vi "Elevator PID.vi"(2 "error in":errorcluster, 3 "PID gains":T1={"proportional gain (Kc)"=0.01, "integral time (Ti, min)"=0.0, "derivative time (Td, min)"=0.0}, 4 "Position":dbl format="%.2f") -> (0 "error out":errorcluster, 1 "Motor Output":dbl format="%.2f")   [LabVIEW 2018]
uses:
  <vilib>/addons/control/pid/pid.llb/PID (DBL).vi
  <vilib>/addons/control/pid/NI_PID_pid.lvlib
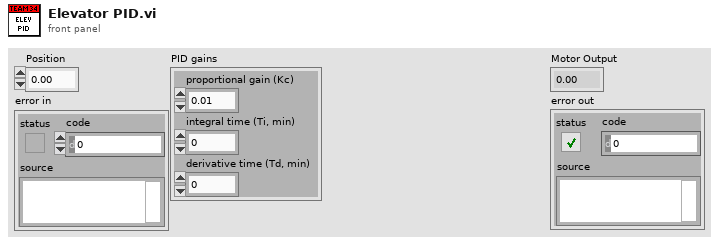
[diagram p1: front panel]
types:
  T1 = cluster{"proportional gain (Kc)":dbl, "integral time (Ti, min)":dbl, "derivative time (Td, min)":dbl}
  T2 = typedef "WPI_EncoderDevRef.ctl" = cluster{"DevStatus":errorcluster, "EncoderIndex":T3, "CounterIndex":T4, "DistancePerCount":dbl, "Decoding Type":T5}
  T3 = typedef "FPGA_EncoderIdx.ctl" = enum8{"Enc 0", "Enc 1", "Enc 2", "Enc 3", "Enc 4", "Enc 5", "Enc 6", "Enc 7", "Invalid"}
  T4 = typedef "FPGA_CounterCtrSystemIndex.ctl" = enum8{"Ctr 0", "Ctr 1", "Ctr 2", "Ctr 3", "Ctr 4", "Ctr 5", "Ctr 6", "Ctr 7", "Invalid"}
  T5 = typedef "WPI_EncoderType.ctl" = enum16{"1x", "2x", "4x"}
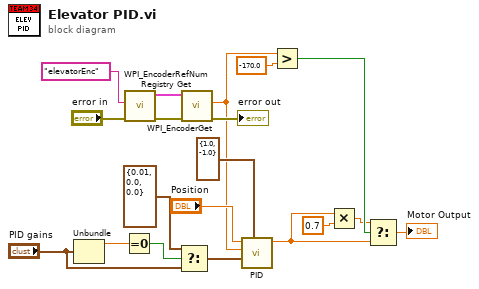
[diagram p0: block diagram]
diagram:
  n1 = Unbundle("PID gains") -> ("proportional gain (Kc)"=w13:dbl)  [unwired: 2 out]
  n2 = Equal To 0?(x=w13) -> (x = 0?=w10:bool)
  n3 = call <vilib>:"WPI_EncoderRefNum Registry Get.vi"("error in (no error)"="error in", "refnum name"="elevatorEnc") -> ("error out"=w15:errorcluster, "EncoderDevRef"=w18:T2)  [unwired: 8 in]
  n4 = Select(t=T1 {"proportional gain (Kc)"=0.01, "integral time (Ti, min)"=0.0, "derivative time (Td, min)"=0.0} ("PID gains"), s=w10, f="PID gains") -> (s? t:f=w11:T1)
  n5 = call <vilib>:"WPI_EncoderGet.vi"("error in (no error)"=w15, "EncoderDevRef"=w18) -> ("error out"=→"error out":errorcluster, "Distance"=w7:dbl)  [unwired: 4 in, 4 out]
  n6 = call-poly <vilib>:"PID.vi"("output range"=cluster{"output high":dbl, "output low":dbl} {"output high"=1.0, "output low"=-1.0}, "PID gains"=w11, "process variable"=w7, "setpoint"="Position") -> ("output"=w1:dbl)  [unwired: 6 in, 1 out]
  n7 = Greater?(x=w7, y=-170.0) -> (0:w4:bool)
  n8 = Multiply(x=w1, y=0.7) -> (x*y=w3:dbl)
  n9 = Select(t=w3, s=w4, f=w1) -> (s? t:f=→"Motor Output":dbl)
